vi "Thread dispatchor.vi"(6 "open fp?":bool, 8 "error in (no error)":errorcluster, 11 "Numeric":i32) -> (0 "error out":errorcluster)   [LabVIEW 2020]
uses:
  df1e56f2-ad5a-4bca-bc92-1cfc5d19beee.vi
  fb37dcd6-ea99-4d19-9594-8912ef1d6254.vi
  <vilib>/Utility/error.llb/Clear Errors.vi
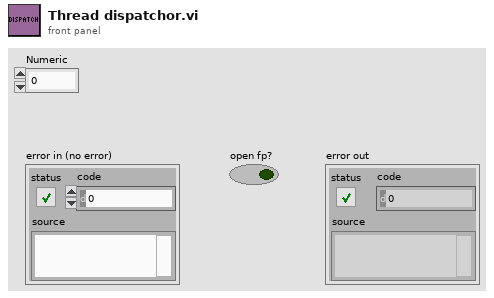
[diagram p1: front panel]
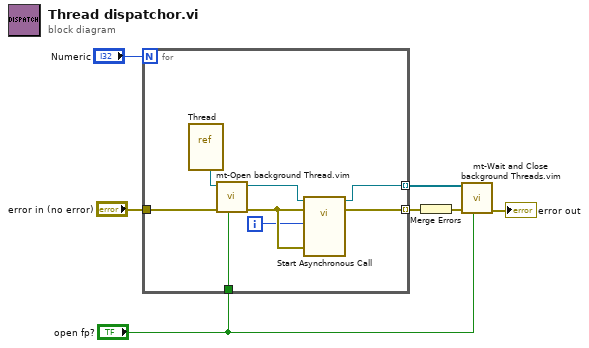
[diagram p0: block diagram]
diagram:
  n1 = for {
    N: "Numeric" -> [_]
    tunnel: [w10] -> w7 mode=indexing
    tunnel: [w12] -> w6 mode=indexing
    tunnel: "error in (no error)" -> [w14]
    tunnel: "open fp?" -> [w13]
    i -> [w8]
    n2 = vi-ref "Thread.vi"() -> (w15:refnum<vi>)
    n3 = call "mt-Open background Thread.vim"("open fp?"=w13, "error in (no error)"=w14, "tempate"=w15) -> ("error out"=w9:errorcluster, "VI out"=w11:refnum<vi>)  [unwired: 7 in]
    n4 = call-by-ref "Start Asynchronous Call"(reference=w11, error in=w9, "Error in"=w9, "indicator 2"=w8) -> (reference out=w10:refnum<vi>, error out=w12:errorcluster)  [unwired: 9 in, 1 out]
  }
  n5 = Merge Errors(w6) -> (w5:errorcluster)
  n6 = call "mt-Wait and Close background Threads.vim"("open fp?"="open fp?", "error in (no error)"=w5, "Array"=w7) -> ("error out"=→"error out":errorcluster)  [unwired: 8 in]
